vi "VI.vi"(0 "X":dbl, 1 "Y":dbl) -> (7 "Result":dbl)   [LabVIEW 2023]
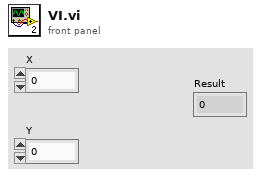
[diagram p1: front panel]
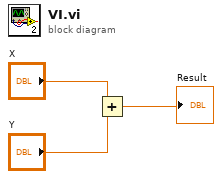
[diagram p0: block diagram]
diagram:
  n1 = Add(x="X", y="Y") -> (x+y=→"Result":dbl)
